vi "plugins_run.vi"(8 "Error In":errorcluster, 10 "Plugin Index":u16, 11 "Plugins In":T1(array[cluster])) -> (0 "Error Out":errorcluster, 3 "Plugins":T1(array[cluster]))   [LabVIEW 2015]
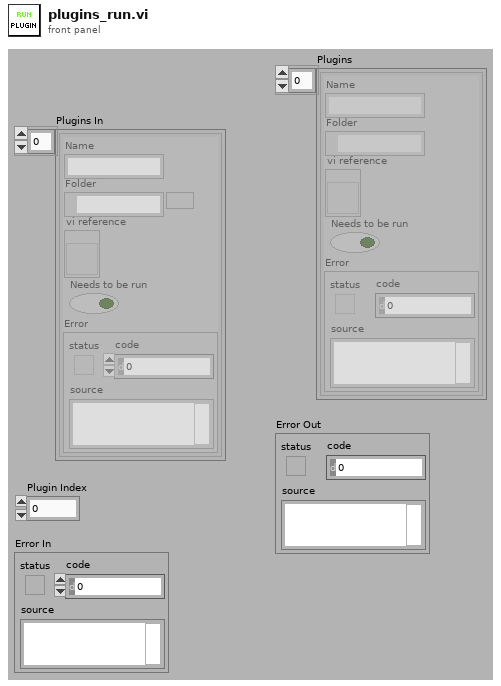
[diagram p1: front panel]
types:
  T1 = cluster{"Name":string, "Folder":path, "vi reference":refnum<vi>, "Needs to be run":bool, "Error":errorcluster}[]
  T2 = cluster{"Name":string, "Folder":path, "vi reference":refnum<vi>, "Needs to be run":bool, "Error":errorcluster}
  T3 = enum32{"Bad", "Idle", "Run top level", "Running"}
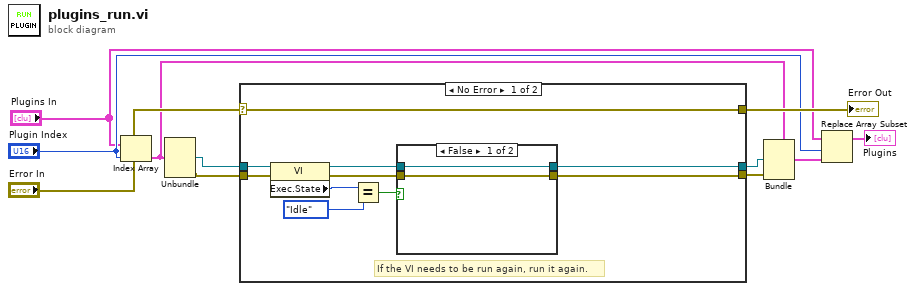
[diagram p0: block diagram]
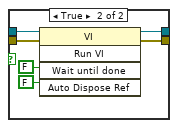
[diagram p2: hidden frame]
diagram:
  n1 = Index Array(array="Plugins In", index="Plugin Index") -> (element=w6:T2)
  n2 = Unbundle(w6) -> ("vi reference"=w1:refnum<vi>, "Error"=w2:errorcluster)  [unwired: 3 out]
  n3 = case shown="No Error" "Error In" {
    selector: "Error In" -> [w12 w30]
    tunnel: [w16 w31] -> w5
    tunnel: w1 -> [w15 w31]
    tunnel: w2 -> [w14 w32]
    tunnel: [w13 w32] -> w4
    tunnel: [w12 w30] -> w10
    frame No Error {
      # "If the VI needs to be run again, run it again."
      n4 = property class="VI"(reference=w15, error in=w14) -> (reference out=w19:refnum<vi>, error out=w18:errorcluster, "Exec.State"=w21:T3)
      n5 = Equal?(x=w21, y=T3."Idle" ("x")) -> (x = y?=w17:bool)
      n6 = case shown="False" w17 {
        tunnel: w19 -> [w23 w29]
        tunnel: w18 -> [w22 w28]
        tunnel: [w23 w25] -> w16
        tunnel: [w22 w24] -> w13
        frame False {
        }
        frame True {
          n7 = invoke class="VI" method="Run VI"(reference=w29, error in=w28, "Wait until done"=FALSE ("Wait Until Done"), "Auto Dispose Ref"=FALSE ("Auto Dispose Reference")) -> (reference out=w25:refnum<vi>, error out=w24:errorcluster)  [unwired: 1 in, 3 out]
        }
      }
    }
    frame Error {
    }
  }
  "Error Out" <- w10
  n8 = Bundle(cluster=w6, "vi reference"=w5, "Error"=w4) -> (w3:T2)  [unwired: 3 in]
  n9 = Replace Array Subset(array="Plugins In", new element=w3, index="Plugin Index") -> (→"Plugins":T1)
